vi "读取分辨率.vi"(0 "DevCfgGet":cluster{"pid":u32, "vid":u32, "ser_num":u64}[](array[cluster]), 5 "设备列表":i32[](array[numeric]), 7 "设备":u16(ring) items=["设备1_22592_3034"], 11 "error in":errorcluster) -> (4 "获取设备信息返回值":i32, 8 "camera_stream_info[]":T1(array[cluster]), 15 "error out":errorcluster)   [LabVIEW 2016]
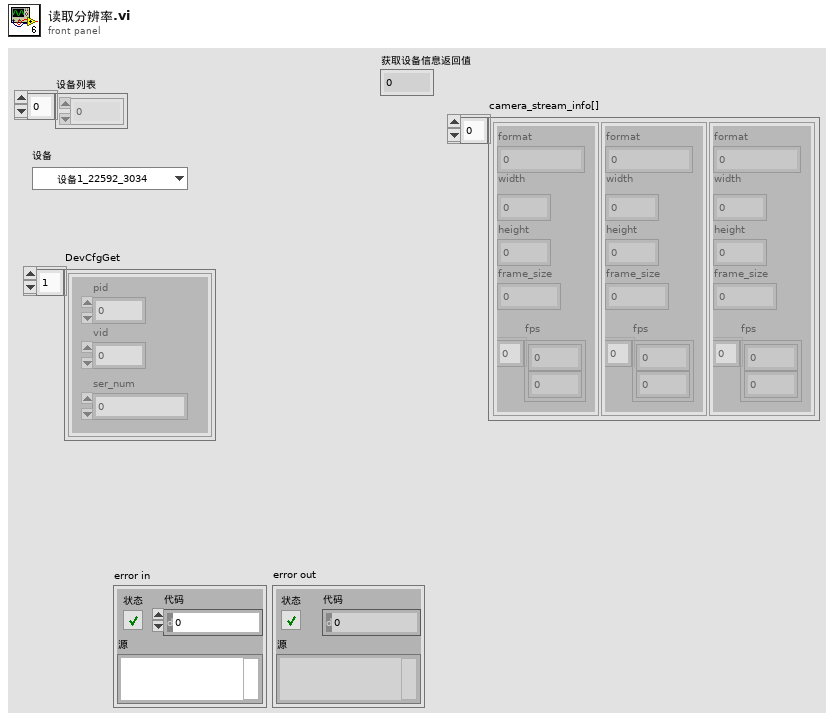
[diagram p1: front panel]
types:
  T1 = cluster{"format":u64, "width":u32, "height":u32, "frame_size":u32, "fps":u32[]}[]
  T2 = cluster{"format":u64, "width":u32, "height":u32, "frame_size":u32, "fps":u32[]}
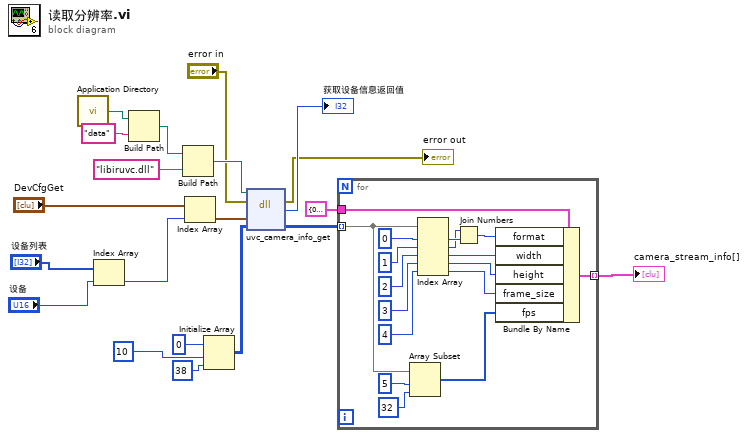
[diagram p0: block diagram]
diagram:
  n1 = call <vilib>:"Application Directory.vi"() -> ("Application Directory"=w17:path)
  n2 = Index Array(array="设备列表", index="设备") -> (element=w10:i32)
  n3 = Build Path(base path=w17, name or relative path="data") -> (appended path=w16:path)
  n4 = Build Path(base path=w16, name or relative path="libiruvc.dll") -> (appended path=w19:path)
  n5 = Index Array(array="DevCfgGet", index=w10) -> (element=w20:cluster{"pid":u32, "vid":u32, "ser_num":u64})
  n6 = Initialize Array(u32 0, 10, 38) -> (w12:u32[][])
  n7 = dll-call lib="D:/libiruvc_0.3.3/windows/x64/dll/libiruvc.dll" fn="uvc_camera_info_get"(path in=w19, error in="error in", "dev_cfg"=w20, "camera_stream_info[]"=w12) -> (error out=→"error out":errorcluster, "return type"=→"获取设备信息返回值":i32, "camera_stream_info[]"=w11:u32[][])  [unwired: 2 in, 1 out]
  n8 = for {
    tunnel: w11 -> [w30] mode=indexing
    tunnel: T2 {"format"=0, "width"=0, "height"=0, "frame_size"=0, "fps"=[]} ("CameraStreamInfo") -> [w29]
    tunnel: [w26] -> w9 mode=indexing
    n9 = Array Subset(array=w30, index=5, length=32) -> (w28:u32[])
    n10 = Index Array(array=w30, index #1=0, index #2=1, index #3=2, index #4=3, index #5=4) -> (element #1=w25:u32, element #2=w24:u32, element #3=w22:u32, element #4=w21:u32, element #5=w27:u32)
    n11 = Join Numbers(hi=w24, lo=w25) -> ((hi.lo)=w23:u64)
    n12 = Bundle By Name(cluster=w29, "format"=w23, "width"=w22, "height"=w21, "frame_size"=w27, "fps"=w28) -> (w26:T2)
  }
  "camera_stream_info[]" <- w9
